vi "_MenuVIs.vi"() -> (3 "VIs":refnum<vi>[](array[refnum]))   [LabVIEW 2017, in "tagdb-UIStateExpr Operations.lvlib"]
uses:
  tagdb-UIStateExpr Operations.lvlib
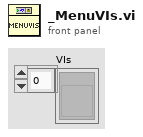
[diagram p1: front panel]
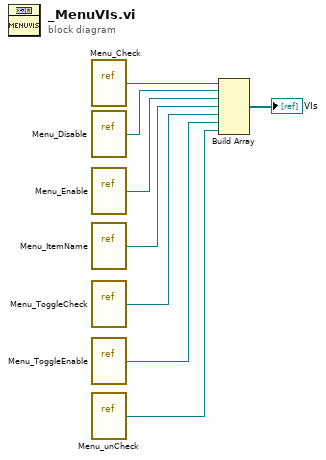
[diagram p0: block diagram]
diagram:
  n1 = vi-ref "Menu_Check.vi"() -> (w3:refnum<vi>)
  n2 = vi-ref "Menu_Disable.vi"() -> (w4:refnum<vi>)
  n3 = vi-ref "Menu_Enable.vi"() -> (w5:refnum<vi>)
  n4 = vi-ref "Menu_ItemName.vi"() -> (w6:refnum<vi>)
  n5 = vi-ref "Menu_ToggleCheck.vi"() -> (w7:refnum<vi>)
  n6 = vi-ref "Menu_ToggleEnable.vi"() -> (w8:refnum<vi>)
  n7 = vi-ref "Menu_unCheck.vi"() -> (w2:refnum<vi>)
  n8 = Build Array(w3, w4, w5, w6, w7, w8, w2) -> (→"VIs":refnum<vi>[])
